vi "Discharge_Loop_VI.vi"() -> ()   [LabVIEW 2017]
uses:
  <vilib>/Plasmionique/MB Master/MB_Master_TCP/MB_Master_TCP.lvclass
  <vilib>/Plasmionique/MB Master/MB Master.lvlib
  C:/Program Files (x86)/National Instruments/LabVIEW 2017/vi.lib/Plasmionique/MB Master/MB_Master/MB_Master.lvclass
panel:
  out "BMS 2 IP Address":string
  out "Inverter 2 IP Address":string
  out "Inverter 1 IP Address":string
  out "BMS 1 IP Address":string
  out "SEL IP Address":string
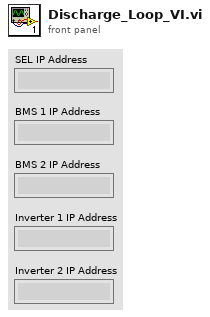
[diagram p1: front panel]
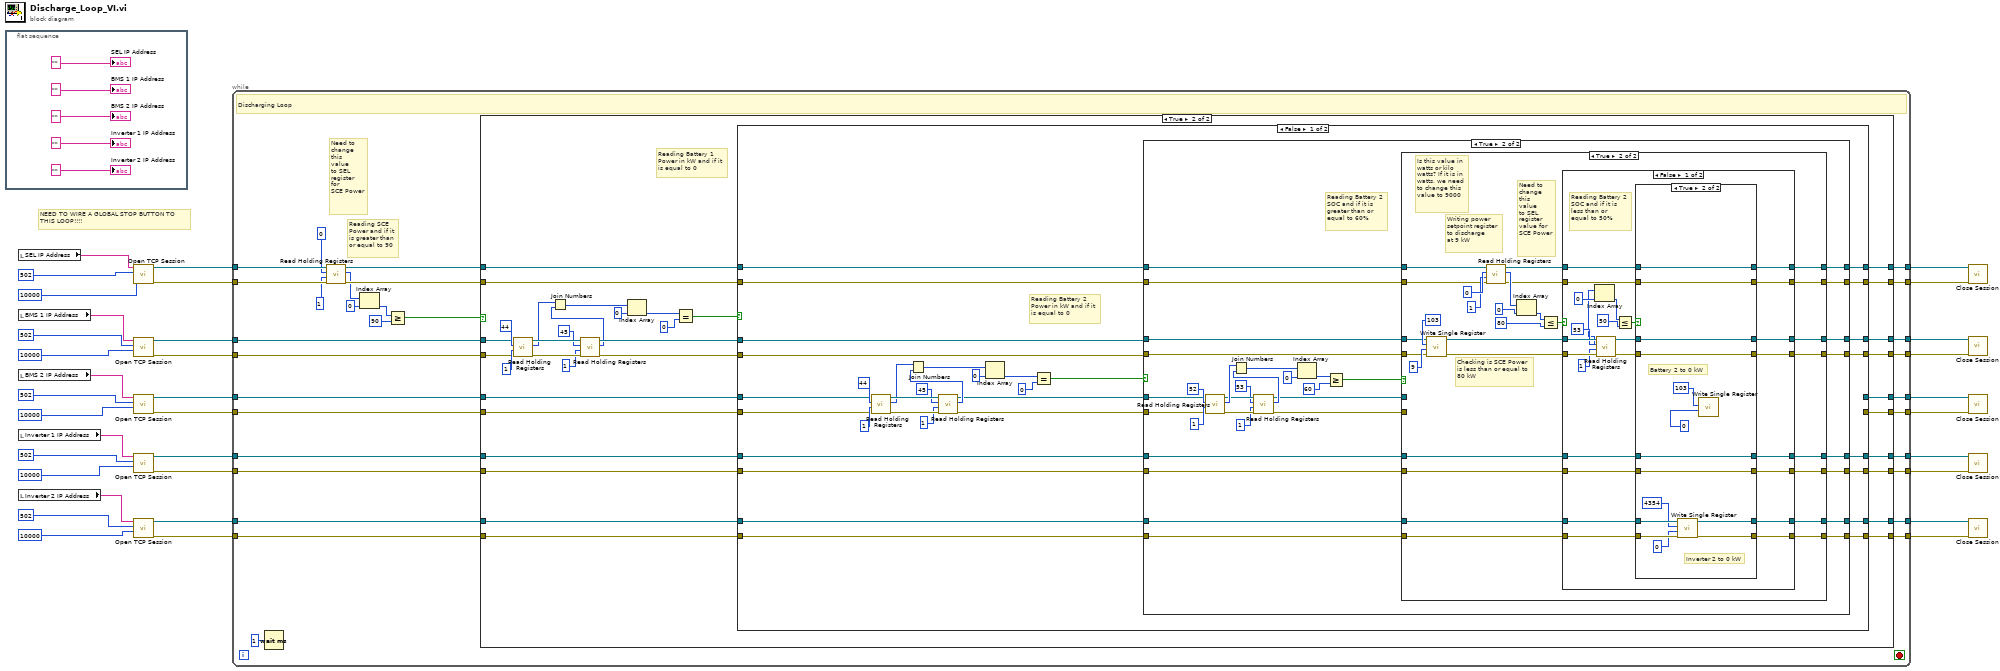
[diagram p0: block diagram]
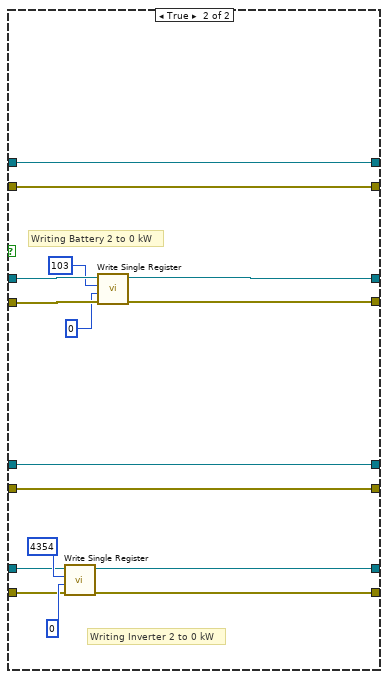
[diagram p6: hidden frame]
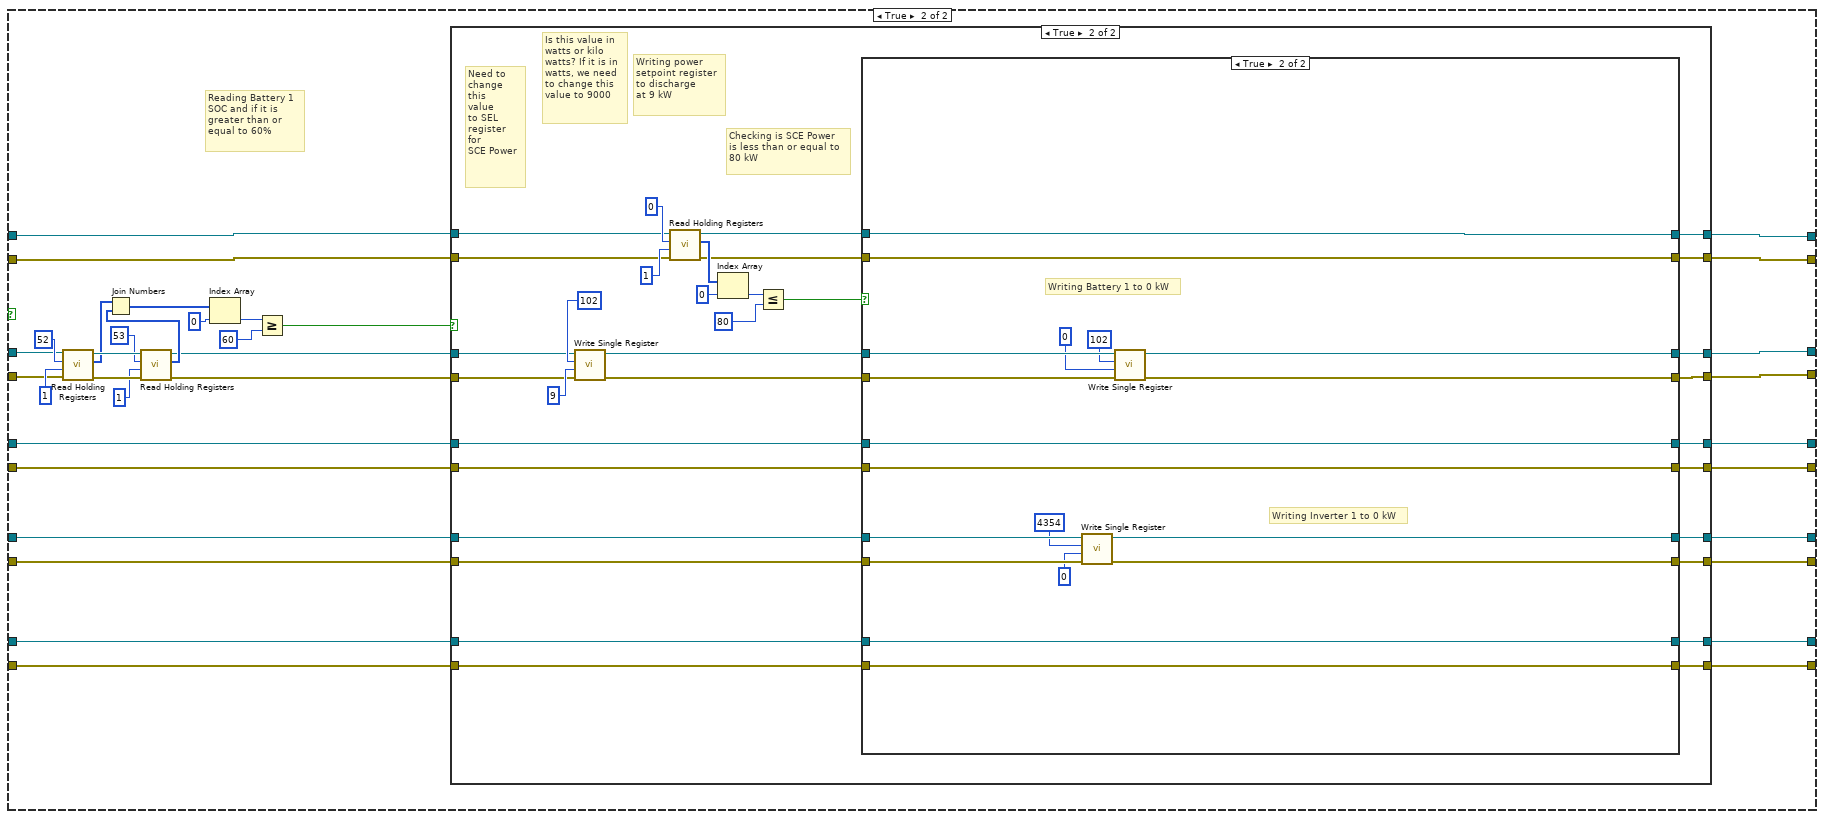
[diagram p7: hidden frame]
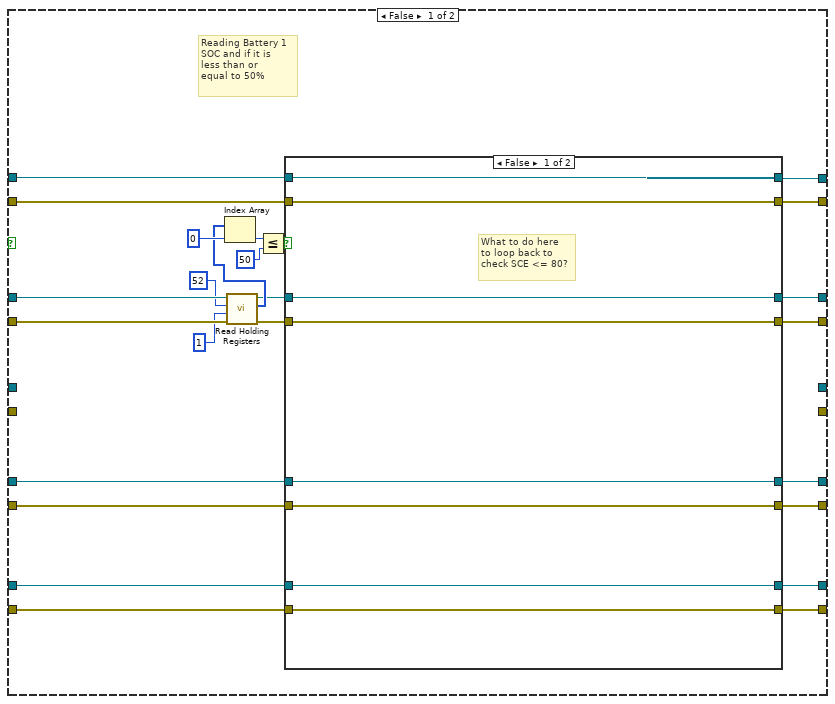
[diagram p9: hidden frame]
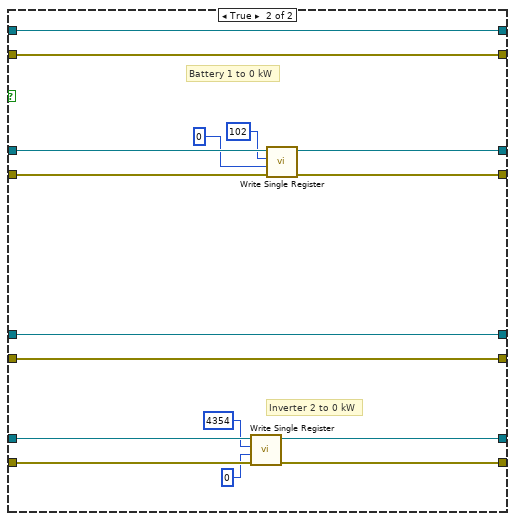
[diagram p10: hidden frame]
diagram:
  # "NEED TO WIRE A GLOBAL STOP BUTTON TO \nTHIS LOOP!!!!"
  n1 = flat-sequence {
    frame #0 {
      "SEL IP Address" <- ""
      "BMS 1 IP Address" <- ""
      "Inverter 1 IP Address" <- ""
      "Inverter 2 IP Address" <- ""
      "BMS 2 IP Address" <- ""
    }
  }
  n2 = local read "SEL IP Address"() -> (w33:string)
  n3 = local read "BMS 1 IP Address"() -> (w26:string)
  n4 = local read "BMS 2 IP Address"() -> (w7:string)
  n5 = local read "Inverter 1 IP Address"() -> (w23:string)
  n6 = local read "Inverter 2 IP Address"() -> (w20:string)
  n7 = call <vilib>:"Open TCP Session.vi"("Timeout (10000)"=10000, "Port (502)"=u16 502, "IP Address"=w33) -> ("error out"=w31:errorcluster, "MB_TCP session"=w32:refnum<class "MB_Master_TCP.lvclass">)  [unwired: 7 in]
  n8 = call <vilib>:"Open TCP Session.vi"("Timeout (10000)"=10000, "Port (502)"=u16 502, "IP Address"=w26) -> ("error out"=w29:errorcluster, "MB_TCP session"=w30:refnum<class "MB_Master_TCP.lvclass">)  [unwired: 7 in]
  n9 = call <vilib>:"Open TCP Session.vi"("Timeout (10000)"=10000, "Port (502)"=u16 502, "IP Address"=w7) -> ("error out"=w3:errorcluster, "MB_TCP session"=w4:refnum<class "MB_Master_TCP.lvclass">)  [unwired: 7 in]
  n10 = call <vilib>:"Open TCP Session.vi"("Timeout (10000)"=10000, "Port (502)"=u16 502, "IP Address"=w23) -> ("error out"=w27:errorcluster, "MB_TCP session"=w28:refnum<class "MB_Master_TCP.lvclass">)  [unwired: 7 in]
  n11 = call <vilib>:"Open TCP Session.vi"("Timeout (10000)"=10000, "Port (502)"=u16 502, "IP Address"=w20) -> ("error out"=w16:errorcluster, "MB_TCP session"=w17:refnum<class "MB_Master_TCP.lvclass">)  [unwired: 7 in]
  n12 = while {
    tunnel: w32 -> [w69]
    tunnel: w31 -> [w70]
    tunnel: [w59] -> w15
    tunnel: [w58] -> w14
    tunnel: w30 -> [w56]
    tunnel: w29 -> [w55]
    tunnel: w28 -> [w54]
    tunnel: w27 -> [w53]
    tunnel: w17 -> [w52]
    tunnel: w16 -> [w51]
    tunnel: [w50] -> w13
    tunnel: [w49] -> w12
    tunnel: [w48] -> w11
    tunnel: [w47] -> w10
    tunnel: [w46] -> w9
    tunnel: [w45] -> w8
    tunnel: w4 -> [w44]
    tunnel: w3 -> [w43]
    tunnel: [w42] -> w1
    tunnel: [w41] -> w2
    stop <- _ stop-if-true
    # "Reading SCE\nPower and if it\nis greater than \nor equal to 90"
    # "Need to \nchange \nthis \nvalue\nto SEL \nregister \nfor \nSCE Power"
    # "Discharging Loop"
    n13 = Wait (ms)(milliseconds to wait=u32 1) -> ()  [unwired: 1 out]
    n14 = call <vilib>:"Read Holding Registers.vi"("error in (no error)"=w70, "quantity"=u16 1, "starting address"=u16 0, "MB session in"=w69) -> ("error out"=w65:errorcluster, "Registers"=w64:u16[], "MB session out"=w66:refnum<class "MB_Master_TCP.lvclass">)  [unwired: 5 in]
    n15 = Index Array(array=w64, index=0) -> (element=w62:u16)
    n16 = Greater Or Equal?(x=w62, y=u16 90) -> (x >= y?=w60:bool)
    n17 = case shown="True" w60 {
      tunnel: w66 -> [w80 w111]
      tunnel: w65 -> [w79 w110]
      tunnel: [w80 w105] -> w59
      tunnel: [w79 w104] -> w58
      tunnel: w56 -> [w78 w113]
      tunnel: w55 -> [w77 w112]
      tunnel: w54 -> [w76 w109]
      tunnel: w53 -> [w75 w108]
      tunnel: w52 -> [w74 w107]
      tunnel: w51 -> [w73 w106]
      tunnel: [w78 w103] -> w50
      tunnel: [w77 w102] -> w49
      tunnel: [w76 w101] -> w48
      tunnel: [w75 w100] -> w47
      tunnel: [w74 w99] -> w46
      tunnel: [w73 w98] -> w45
      tunnel: w44 -> [w72 w84]
      tunnel: w43 -> [w71 w83]
      tunnel: [w72 w82] -> w42
      tunnel: [w71 w81] -> w41
      frame False {
      }
      frame True {
        # "Reading Battery 1\nPower in kW and if it\nis equal to 0"
        n18 = call <vilib>:"Read Holding Registers.vi"("error in (no error)"=w112, "quantity"=u16 1, "starting address"=u16 44, "MB session in"=w113) -> ("error out"=w96:errorcluster, "Registers"=w90:u16[], "MB session out"=w97:refnum<class "MB_Master_TCP.lvclass">)  [unwired: 5 in]
        n19 = call <vilib>:"Read Holding Registers.vi"("error in (no error)"=w96, "quantity"=u16 1, "starting address"=u16 45, "MB session in"=w97) -> ("error out"=w92:errorcluster, "Registers"=w91:u16[], "MB session out"=w93:refnum<class "MB_Master_TCP.lvclass">)  [unwired: 5 in]
        n20 = Join Numbers(hi=w90, lo=w91) -> ((hi.lo)=w89:u32[])
        n21 = Index Array(array=w89, index=0) -> (element=w87:u32)
        n22 = Equal?(x=w87, y=u32 0) -> (x = y?=w85:bool)
        n23 = case shown="False" w85 {
          tunnel: w111 -> [w148 w318]
          tunnel: w110 -> [w147 w317]
          tunnel: w93 -> [w134 w320]
          tunnel: w92 -> [w133 w319]
          tunnel: w109 -> [w146 w316]
          tunnel: w108 -> [w145 w315]
          tunnel: w107 -> [w144 w314]
          tunnel: w106 -> [w143 w313]
          tunnel: [w142 w312] -> w105
          tunnel: [w141 w311] -> w104
          tunnel: [w140 w310] -> w103
          tunnel: [w139 w309] -> w102
          tunnel: [w138 w308] -> w101
          tunnel: [w137 w307] -> w100
          tunnel: [w136 w306] -> w99
          tunnel: [w135 w305] -> w98
          tunnel: w84 -> [w120 w304]
          tunnel: w83 -> [w119 w303]
          tunnel: [_ w289] -> w82
          tunnel: [_ w288] -> w81
          frame False {
            # "Reading Battery 2\nPower in kW and if it\nis equal to 0"
            n24 = call <vilib>:"Read Holding Registers.vi"("error in (no error)"=w119, "quantity"=u16 1, "starting address"=u16 44, "MB session in"=w120) -> ("error out"=w129:errorcluster, "Registers"=w125:u16[], "MB session out"=w130:refnum<class "MB_Master_TCP.lvclass">)  [unwired: 5 in]
            n25 = call <vilib>:"Read Holding Registers.vi"("error in (no error)"=w129, "quantity"=u16 1, "starting address"=u16 45, "MB session in"=w130) -> ("error out"=w117:errorcluster, "Registers"=w126:u16[], "MB session out"=w118:refnum<class "MB_Master_TCP.lvclass">)  [unwired: 5 in]
            n26 = Join Numbers(hi=w125, lo=w126) -> ((hi.lo)=w124:u32[])
            n27 = Index Array(array=w124, index=0) -> (element=w122:u32)
            n28 = Equal?(x=w122, y=u32 0) -> (x = y?=w116:bool)
            n29 = case shown="True" w116 {
              tunnel: w148 -> [w156 w188]
              tunnel: w147 -> [w155 w189]
              tunnel: w134 -> [w154 w175]
              tunnel: w133 -> [w153 w174]
              tunnel: w146 -> [w152 w187]
              tunnel: w145 -> [w151 w186]
              tunnel: w144 -> [w150 w185]
              tunnel: w143 -> [w149 w184]
              tunnel: [w156 w183] -> w142
              tunnel: [w155 w182] -> w141
              tunnel: [w154 w181] -> w140
              tunnel: [w153 w180] -> w139
              tunnel: [w152 w179] -> w138
              tunnel: [w151 w178] -> w137
              tunnel: [w150 w177] -> w136
              tunnel: [w149 w176] -> w135
              tunnel: w118 -> [_ w161]
              tunnel: w117 -> [_ w160]
              frame False {
              }
              frame True {
                # "Reading Battery 2 \nSOC and if it is \ngreater than or \nequal to 60%"
                n30 = call <vilib>:"Read Holding Registers.vi"("error in (no error)"=w160, "quantity"=u16 1, "starting address"=u16 52, "MB session in"=w161) -> ("error out"=w169:errorcluster, "Registers"=w170:u16[], "MB session out"=w168:refnum<class "MB_Master_TCP.lvclass">)  [unwired: 5 in]
                n31 = call <vilib>:"Read Holding Registers.vi"("error in (no error)"=w169, "quantity"=u16 1, "starting address"=u16 53, "MB session in"=w168) -> ("error out"=w157:errorcluster, "Registers"=w171:u16[], "MB session out"=w158:refnum<class "MB_Master_TCP.lvclass">)  [unwired: 5 in]
                n32 = Join Numbers(hi=w170, lo=w171) -> ((hi.lo)=w172:u32[])
                n33 = Index Array(array=w172, index=0) -> (element=w173:u32)
                n34 = Greater Or Equal?(x=w173, y=u32 60) -> (x >= y?=w159:bool)
                n35 = case shown="True" w159 {
                  tunnel: w188 -> [w195 w213]
                  tunnel: w189 -> [w194 w212]
                  tunnel: w175 -> [_ w211]
                  tunnel: w174 -> [_ w210]
                  tunnel: w187 -> [w193 w207]
                  tunnel: w186 -> [w192 w206]
                  tunnel: w185 -> [w191 w205]
                  tunnel: w184 -> [w190 w204]
                  tunnel: [w190 w203] -> w176
                  tunnel: [w191 w202] -> w177
                  tunnel: [w192 w201] -> w178
                  tunnel: [w193 w200] -> w179
                  tunnel: [_ w199] -> w180
                  tunnel: [_ w198] -> w181
                  tunnel: [w194 w197] -> w182
                  tunnel: [w195 w196] -> w183
                  tunnel: w158 -> [_ _]
                  tunnel: w157 -> [_ _]
                  frame False {
                  }
                  frame True {
                    # "Checking is SCE Power\nis less than or equal to\n80 kW"
                    # "Need to \nchange \nthis \nvalue\nto SEL \nregister \nvalue for \nSCE Power"
                    # "Writing power\nsetpoint register \nto discharge \nat 9 kW"
                    # "Is this value in \nwatts or kilo \nwatts? If it is in \nwatts, we need \nto change this \nvalue to 9000"
                    n36 = call <vilib>:"Write Single Register.vi"("error in (no error)"=w210, "value"=u16 9, "address"=u16 103, "MB session in"=w211) -> ("error out"=w208:errorcluster, "MB session out"=w209:refnum<class "MB_Master_TCP.lvclass">)  [unwired: 6 in]
                    n37 = call <vilib>:"Read Holding Registers.vi"("error in (no error)"=w212, "quantity"=u16 1, "starting address"=u16 0, "MB session in"=w213) -> ("error out"=w214:errorcluster, "Registers"=w220:u16[], "MB session out"=w215:refnum<class "MB_Master_TCP.lvclass">)  [unwired: 5 in]
                    n38 = Index Array(array=w220, index=0) -> (element=w218:u16)
                    n39 = Less Or Equal?(x=w218, y=u16 80) -> (x <= y?=w216:bool)
                    n40 = case shown="False" w216 {
                      tunnel: w215 -> [w240 w285]
                      tunnel: w214 -> [w239 w284]
                      tunnel: w209 -> [w248 w283]
                      tunnel: w208 -> [w249 w282]
                      tunnel: w207 -> [w236 w273]
                      tunnel: w206 -> [w235 w272]
                      tunnel: [w234 w285] -> w196
                      tunnel: [w233 w284] -> w197
                      tunnel: [w232 w279] -> w198
                      tunnel: [w231 w278] -> w199
                      tunnel: [w228 w273] -> w200
                      tunnel: [w227 w272] -> w201
                      tunnel: w205 -> [w230 w277]
                      tunnel: w204 -> [w229 w276]
                      tunnel: [w226 w275] -> w202
                      tunnel: [w225 w274] -> w203
                      frame False {
                        # "Reading Battery 2 \nSOC and if it is \nless than or \nequal to 50%"
                        n41 = call <vilib>:"Read Holding Registers.vi"("error in (no error)"=w249, "quantity"=u16 1, "starting address"=u16 53, "MB session in"=w248) -> ("error out"=w237:errorcluster, "Registers"=w242:u16[], "MB session out"=w238:refnum<class "MB_Master_TCP.lvclass">)  [unwired: 5 in]
                        n42 = Index Array(array=w242, index=0) -> (element=w244:u16)
                        n43 = Less Or Equal?(x=w244, y=u16 50) -> (x <= y?=w241:bool)
                        n44 = case shown="True" w241 {
                          tunnel: w240 -> [w250 w271]
                          tunnel: w239 -> [w251 w270]
                          tunnel: w238 -> [w257 w259]
                          tunnel: w237 -> [w256 w258]
                          tunnel: w236 -> [w255 w267]
                          tunnel: w235 -> [w254 w266]
                          tunnel: [w250 w271] -> w234
                          tunnel: [w251 w270] -> w233
                          tunnel: [w257 w259] -> w232
                          tunnel: [w256 w258] -> w231
                          tunnel: w230 -> [w253 w265]
                          tunnel: w229 -> [w252 w264]
                          tunnel: [w255 w267] -> w228
                          tunnel: [w254 w266] -> w227
                          tunnel: [w253 w263] -> w226
                          tunnel: [w252 w262] -> w225
                          frame False {
                            # "What to do here \nto loop back to \ncheck SCE <= 80?"
                          }
                          frame True {
                            # "Inverter 2 to 0 kW"
                            # "Battery 2 to 0 kW"
                            n45 = call <vilib>:"Write Single Register.vi"("error in (no error)"=w264, "value"=u16 0, "address"=u16 4354, "MB session in"=w265) -> ("error out"=w262:errorcluster, "MB session out"=w263:refnum<class "MB_Master_TCP.lvclass">)  [unwired: 6 in]
                            n46 = call <vilib>:"Write Single Register.vi"("value"=u16 0, "address"=u16 103) -> ()  [unwired: 8 in, 2 out]
                          }
                        }
                      }
                      frame True {
                        # "Writing Inverter 2 to 0 kW"
                        # "Writing Battery 2 to 0 kW"
                        n47 = call <vilib>:"Write Single Register.vi"("error in (no error)"=w276, "value"=u16 0, "address"=u16 4354, "MB session in"=w277) -> ("error out"=w274:errorcluster, "MB session out"=w275:refnum<class "MB_Master_TCP.lvclass">)  [unwired: 6 in]
                        n48 = call <vilib>:"Write Single Register.vi"("error in (no error)"=w282, "value"=u16 0, "address"=u16 103, "MB session in"=w283) -> ("error out"=w278:errorcluster, "MB session out"=w279:refnum<class "MB_Master_TCP.lvclass">)  [unwired: 6 in]
                      }
                    }
                  }
                }
              }
            }
          }
          frame True {
            # "Reading Battery 1 \nSOC and if it is \ngreater than or \nequal to 60%"
            n49 = call <vilib>:"Read Holding Registers.vi"("error in (no error)"=w319, "quantity"=u16 1, "starting address"=u16 52, "MB session in"=w320) -> ("error out"=w301:errorcluster, "Registers"=w298:u16[], "MB session out"=w302:refnum<class "MB_Master_TCP.lvclass">)  [unwired: 5 in]
            n50 = call <vilib>:"Read Holding Registers.vi"("error in (no error)"=w301, "quantity"=u16 1, "starting address"=u16 53, "MB session in"=w302) -> ("error out"=w295:errorcluster, "Registers"=w297:u16[], "MB session out"=w296:refnum<class "MB_Master_TCP.lvclass">)  [unwired: 5 in]
            n51 = Join Numbers(hi=w298, lo=w297) -> ((hi.lo)=w293:u32[])
            n52 = Index Array(array=w293, index=0) -> (element=w292:u32)
            n53 = Greater Or Equal?(x=w292, y=u32 60) -> (x >= y?=w290:bool)
            n54 = case shown="True" w290 {
              tunnel: w318 -> [_ w344]
              tunnel: w317 -> [_ w343]
              tunnel: w296 -> [_ w342]
              tunnel: w295 -> [_ w341]
              tunnel: w316 -> [_ w338]
              tunnel: w315 -> [_ w337]
              tunnel: w314 -> [_ w336]
              tunnel: w313 -> [_ w335]
              tunnel: [_ w334] -> w305
              tunnel: [_ w333] -> w306
              tunnel: [_ w332] -> w307
              tunnel: [_ w331] -> w308
              tunnel: [_ w330] -> w309
              tunnel: [_ w329] -> w310
              tunnel: [_ w328] -> w311
              tunnel: [_ w327] -> w312
              tunnel: w304 -> [_ w326]
              tunnel: w303 -> [_ w325]
              tunnel: [_ w324] -> w289
              tunnel: [_ w323] -> w288
              frame False {
              }
              frame True {
                # "Checking is SCE Power\nis less than or equal to\n80 kW"
                # "Need to \nchange \nthis \nvalue\nto SEL \nregister \nfor \nSCE Power"
                # "Writing power\nsetpoint register \nto discharge \nat 9 kW"
                # "Is this value in \nwatts or kilo \nwatts? If it is in \nwatts, we need \nto change this \nvalue to 9000"
                n55 = call <vilib>:"Write Single Register.vi"("error in (no error)"=w341, "value"=u16 9, "address"=u16 102, "MB session in"=w342) -> ("error out"=w339:errorcluster, "MB session out"=w340:refnum<class "MB_Master_TCP.lvclass">)  [unwired: 6 in]
                n56 = call <vilib>:"Read Holding Registers.vi"("error in (no error)"=w343, "quantity"=u16 1, "starting address"=u16 0, "MB session in"=w344) -> ("error out"=w345:errorcluster, "Registers"=w351:u16[], "MB session out"=w346:refnum<class "MB_Master_TCP.lvclass">)  [unwired: 5 in]
                n57 = Index Array(array=w351, index=0) -> (element=w349:u16)
                n58 = Less Or Equal?(x=w349, y=u16 80) -> (x <= y?=w347:bool)
                n59 = case shown="True" w347 {
                  tunnel: w346 -> [w371 w418]
                  tunnel: w345 -> [w370 w417]
                  tunnel: w340 -> [w379 w416]
                  tunnel: w339 -> [w380 w415]
                  tunnel: w338 -> [w367 w422]
                  tunnel: w337 -> [w366 w421]
                  tunnel: [w365 w418] -> w327
                  tunnel: [w364 w417] -> w328
                  tunnel: [w363 w412] -> w329
                  tunnel: [w362 w411] -> w330
                  tunnel: [w359 w410] -> w331
                  tunnel: [w358 w409] -> w332
                  tunnel: w336 -> [w361 w406]
                  tunnel: w335 -> [w360 w405]
                  tunnel: [w357 w406] -> w333
                  tunnel: [w356 w405] -> w334
                  tunnel: w326 -> [_ w408]
                  tunnel: w325 -> [_ w407]
                  tunnel: [_ w408] -> w324
                  tunnel: [_ w407] -> w323
                  frame False {
                    # "Reading Battery 1 \nSOC and if it is \nless than or \nequal to 50%"
                    n60 = call <vilib>:"Read Holding Registers.vi"("error in (no error)"=w380, "quantity"=u16 1, "starting address"=u16 52, "MB session in"=w379) -> ("error out"=w368:errorcluster, "Registers"=w373:u16[], "MB session out"=w369:refnum<class "MB_Master_TCP.lvclass">)  [unwired: 5 in]
                    n61 = Index Array(array=w373, index=0) -> (element=w375:u16)
                    n62 = Less Or Equal?(x=w375, y=u16 50) -> (x <= y?=w372:bool)
                    n63 = case shown="False" w372 {
                      tunnel: w371 -> [w381 w404]
                      tunnel: w370 -> [w382 w403]
                      tunnel: w369 -> [w388 w401]
                      tunnel: w368 -> [w387 w402]
                      tunnel: w367 -> [w386 w396]
                      tunnel: w366 -> [w385 w395]
                      tunnel: [w381 w404] -> w365
                      tunnel: [w382 w403] -> w364
                      tunnel: [w388 w400] -> w363
                      tunnel: [w387 w399] -> w362
                      tunnel: w361 -> [w384 w394]
                      tunnel: w360 -> [w383 w393]
                      tunnel: [w386 w396] -> w359
                      tunnel: [w385 w395] -> w358
                      tunnel: [w384 w392] -> w357
                      tunnel: [w383 w391] -> w356
                      frame False {
                        # "What to do here \nto loop back to \ncheck SCE <= 80?"
                      }
                      frame True {
                        # "Inverter 2 to 0 kW"
                        # "Battery 1 to 0 kW"
                        n64 = call <vilib>:"Write Single Register.vi"("error in (no error)"=w393, "value"=u16 0, "address"=u16 4354, "MB session in"=w394) -> ("error out"=w391:errorcluster, "MB session out"=w392:refnum<class "MB_Master_TCP.lvclass">)  [unwired: 6 in]
                        n65 = call <vilib>:"Write Single Register.vi"("error in (no error)"=w402, "value"=u16 0, "address"=u16 102, "MB session in"=w401) -> ("error out"=w399:errorcluster, "MB session out"=w400:refnum<class "MB_Master_TCP.lvclass">)  [unwired: 6 in]
                      }
                    }
                  }
                  frame True {
                    # "Writing Inverter 1 to 0 kW"
                    # "Writing Battery 1 to 0 kW"
                    n66 = call <vilib>:"Write Single Register.vi"("error in (no error)"=w421, "value"=u16 0, "address"=u16 4354, "MB session in"=w422) -> ("error out"=w409:errorcluster, "MB session out"=w410:refnum<class "MB_Master_TCP.lvclass">)  [unwired: 6 in]
                    n67 = call <vilib>:"Write Single Register.vi"("error in (no error)"=w415, "value"=u16 0, "address"=u16 102, "MB session in"=w416) -> ("error out"=w411:errorcluster, "MB session out"=w412:refnum<class "MB_Master_TCP.lvclass">)  [unwired: 6 in]
                  }
                }
              }
            }
          }
        }
      }
    }
  }
  n68 = call-dynamic "Close Session.vi"("error in (no error)"=w14, "MB TCP session"=w15) -> ()  [unwired: 9 in, 1 out]
  n69 = call-dynamic "Close Session.vi"("error in (no error)"=w12, "MB TCP session"=w13) -> ()  [unwired: 9 in, 1 out]
  n70 = call-dynamic "Close Session.vi"("error in (no error)"=w2, "MB TCP session"=w1) -> ()  [unwired: 9 in, 1 out]
  n71 = call-dynamic "Close Session.vi"("error in (no error)"=w10, "MB TCP session"=w11) -> ()  [unwired: 9 in, 1 out]
  n72 = call-dynamic "Close Session.vi"("error in (no error)"=w8, "MB TCP session"=w9) -> ()  [unwired: 9 in, 1 out]
